vi "read.vi"(8 "error in (no error)":errorcluster, 11 "Temp Control in":refnum<class "Temp Control.lvclass">) -> (0 "error out":errorcluster, 2 "Data":dbl[](array[numeric]), 3 "Temp Control out":refnum<class "Temp Control.lvclass">)   [LabVIEW 2022 SP3, in "Temp Control.lvclass"]
uses:
  Temp Control.lvclass
  Temp Control.lvclass/Temp Control.ctl
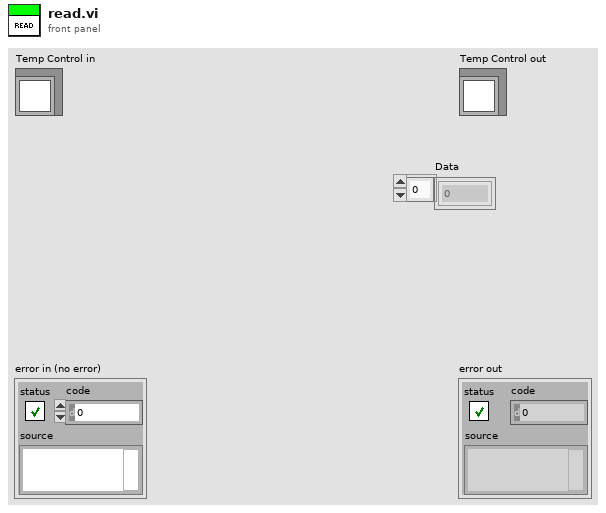
[diagram p1: front panel]
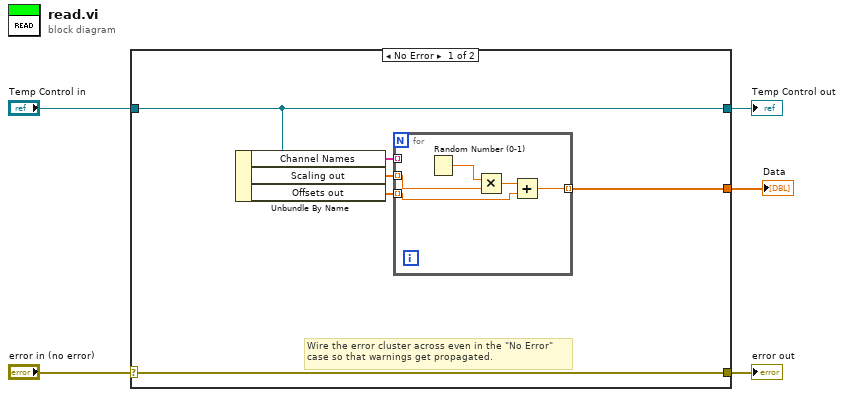
[diagram p0: block diagram]
diagram:
  n1 = case shown="No Error" "error in (no error)" {
    selector: "error in (no error)" -> [w11 w18]
    tunnel: [w11 w18] -> w4
    tunnel: [w10 w17] -> w2
    tunnel: "Temp Control in" -> [w10 w17]
    tunnel: [w8 _] -> w1
    frame No Error {
      # "Wire the error cluster across even in the \"No Error\"\ncase so that warnings get propagated."
      n2 = Unbundle By Name(w10) -> ("Channel Names"=w9:string[], "Scaling out"=w7:dbl[], "Offsets out"=w6:dbl[])
      n3 = for {
        tunnel: w9 -> [_] mode=indexing
        tunnel: [w12] -> w8 mode=indexing
        tunnel: w7 -> [w15] mode=indexing
        tunnel: w6 -> [w13] mode=indexing
        n4 = Random Number (0-1)() -> (number: 0 to 1=w16:dbl)
        n5 = Multiply(x=w16, y=w15) -> (x*y=w14:dbl)
        n6 = Add(x=w14, y=w13) -> (x+y=w12:dbl)
      }
    }
    frame Error {
    }
  }
  "error out" <- w4
  "Temp Control out" <- w2
  "Data" <- w1
